vi "Fc_create_MenuSelections.vi"(8 "error in (no error)":errorcluster, 11 "Menu in":refnum<k9>) -> (0 "error out":errorcluster)   [LabVIEW 2021]
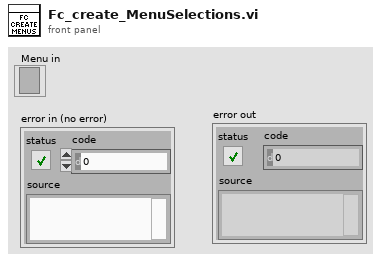
[diagram p1: front panel]
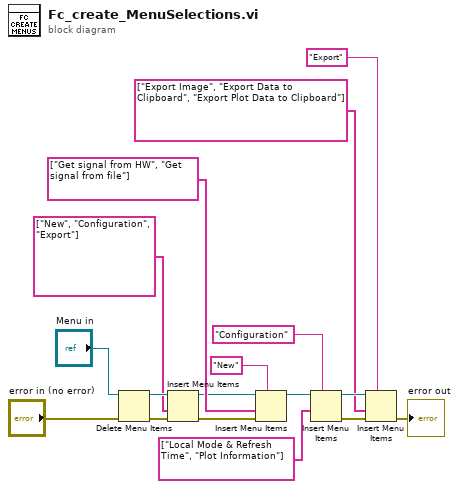
[diagram p0: block diagram]
diagram:
  n1 = Delete Menu Items(6:"error in (no error)", 9:"Menu in") -> (0:w8:errorcluster, 3:w9:refnum<k9>)  [unwired: 2 in]
  n2 = Insert Menu Items(6:w8, 7:string[] ["New", "Configuration", "Export"], 9:w9) -> (0:w2:errorcluster, 3:w3:refnum<k9>)  [unwired: 3 in, 1 out]
  n3 = Insert Menu Items(5:"New", 6:w2, 7:string[] ["Get signal from HW", "Get signal from file"], 9:w3) -> (3:w12:refnum<k9>)  [unwired: 2 in, 2 out]
  n4 = Insert Menu Items(5:"Configuration" ("menu tag"), 7:string[] ["Local Mode & Refresh Time", "Plot Information"] ("item tags"), 9:w12) -> (0:w17:errorcluster, 3:w13:refnum<k9>)  [unwired: 3 in, 1 out]
  n5 = Insert Menu Items(5:"Export" ("menu tag"), 6:w17, 7:string[] ["Export Image", "Export Data to Clipboard", "Export Plot Data to Clipboard"], 9:w13) -> (0:→"error out":errorcluster)  [unwired: 2 in, 2 out]
